vi "Main.vi"() -> ()   [LabVIEW 2025]
doc: "This template is for the Queued Message Handler design pattern.\n\nThe Event Handling Loop generates messages based on user interface actions.\n\nThe Message Handling Loop processes messages generated by the Event Handling Loop, or by other messages. The messages are string values, so new messages can be added easily to the Message Cases case structure in the Message Handling Loop. Each message cluster can also provide an optional value for Message Data, which is a variant that can be converted to whatever message-specific data is required."
uses:
  Public/Controls/CCW button.ctl
  Public/Controls/CW button.ctl
  controls/UI Data.ctl
  support/Message Queue/Enqueue Message (Single).vi
  <vilib>/Utility/error.llb/Error Cluster From Error Code.vi
  <vilib>/ErrorRing/Error Ring.xnode
  support/Message Queue/Message Queue.lvlib
  support/User Event - Stop/User Event - Stop.lvlib
  NI_DAQ/Libraries/NI DAQ/NI DAQ.lvlib
panel:
  in  "Read sensor":bool
  in  "Exit":bool
  in  "Go to zero":bool
  in  "Set zero":bool
  out "Ready":bool caption="Arduino ready"
  out "Save":bool caption="Guardando datos"
  out "Angulo M2":dbl caption="Ángulo \nActual M2" format="%#_3g°"
  out "Angulo M1":dbl caption="Ángulo \nActual M1" format="%#_3g°"
  out "0° M2":bool
  out "0° M1":bool
  in  "RESOLUCIÓN":dbl=1.0 caption="Avance" format="%#_g°"
  in  "CW Button M1":T1
  in  "CCW Button M1":T2
  in  "CCW Button M2":T1
  in  "CW Button M2":T2
  in  "Tab Control":T3(tab)
  out "Valor de Sensor":dbl(slide) scale=0.0..1.0
  in  "Intensidad del Láser":u8(slide) step=1 scale=0.0..255.0
  out "Real Time Measurement":cluster{"X":dbl, "Y":dbl}[](graph)
  in  "Ángulo final":dbl=90.0
  in  "Move motors":bool
  in  "Tiempo (segundos)":dbl=600.0
  in  "Init Fixed Angle":bool
  out "Valor de Sensor 2":dbl(slide) caption="Valor de Sensor" scale=0.0..1.0
  out "Real Time Measurement 2":cluster{"X":dbl, "Y":dbl}[](graph)
  in  "Realizar Análisis":bool
  in  "Abrir Archivo":path
  in  "q Final":dbl=80.0
  in  "q Inicial":dbl=40.0
  out "No. de Muestras":i32
  out "Ancho de Curva":dbl format="%#.3g"
  out "Intensidad \nMáxima":dbl
  out "qR":dbl
  out "Intensidad \nMínima":dbl
  out "q Medio":dbl
  out "Brewster Angle Analysis":cluster{"EJE X":dbl[], dbl[]}(graph)
  out "Índice":dbl
  in  "Abeles Brewster":bool
  in  "Abrir Archivo de Sustrato":path
  in  "Abrir Archivo de Película":path
  in  "calcular error":bool
  out "Abeles Brewster Analysis":cluster{dbl[], dbl[]}[](graph)
  in  "q Inicial 2":dbl=40.0
  in  "q Final  2":dbl=80.0
  out "Película qB":dbl
  out "Película qB +error":dbl
  in  "Error (Grados)":dbl
  out "Sustrato qB":dbl
  out "Sustrato IR":dbl format="%#.4g"
  out "Película IR":dbl format="%#.4g"
  out "ángulo B medio":dbl
  out "Película IR +error":dbl format="%#.4g"
  in  "Cero Maquina":bool
  out "Idle":bool
  in  "Stop motors":bool
  # "Programa: Control de motores a pasos \npara medición de ángulo de Brewster y \ntécnica de Abelès-Brewster"
  # "Desarrollado por: Oscar Javier Silva Hernández &\nDiego Torres Armenta"
  # "Controles Manuales y Automáticos"
  # "MOTOR 1"
  # "MOTOR 2"
  # "Información del sistema"
  # "¡ATENCIÓN! Lea estas instrucciones y recomendaciones antes de operar el programa.\nEste programa ejecuta el control manual y automático del sistema en general.\nUna vez que se haya elegido el puerto COM donde tenemos ubicada nuestra tarjeta de adquisición de datos, el programa inicializará con un protocolo de calibración de motores. NO PRESIONE NINGÚN BOTÓN.\nDe manera automática el programa moverá las platinas rotatorias al ángulo 0°. Una vez que los indicadores 0° M1 y 0° M2 estén encendidos, el indicador del Ángulo Actual M1 se habilitará y el podremos iniciar a operar el programa."
  # "Controles Manuales y Automáticos (Controladores e Indicadores)\n\n-MOTOR 1 & 2: Para ambos motores se tiene un botón de movimiento hacia adelante y otro botón de movimiento hacia atrás indicado con flechas. Durante el reinicio de posición 0°, el botón hacia atrás se deshabilita para evitar conflictos mecánicos.\n-0° M1 & 0° M2: Indicadores de posición 0° para ambos motores.\n-FIN: Indica si se está terminó de realizar un movimiento.\n-Ángulo Actual M1 & M2: Muestra la posición actual para cada motor.\n-RESOLUCIÓN: Valor de grados definido por el usuario para realizar movimientos manuales de manera independiente para cada motor. Es utilizado para alinear el sistema con respecto al láser antes y después de realizar mediciones.\n-Reiniciar Posición: Inicia el protocolo de reinicio de posición para regresar los motores a 0°.\n-Mover y Guardar: Se inicia el barrido ángular desde la posición actual de los motores hasta la posición indicada en el controlador Barrido Angular.\n-Cancelar: Cancela cualquier movimiento o instrucción que se esté ejecutando. My útil para detener instrucciones y cerrar el programa sin tener conflictos."
  # "Parámetros iniciales & Información (Controladores e Indicadores)\n\n-SALIR: Cerramos el programa una vez que hayamos terminado de utilizarlo. Es importante no presionar este botón en medio de un movimiento de motor o alguna otra instrucción.\n-Pantalla: Toda la información generada por los eventos de usuario es mostrada en esta pantalla.\n-Programa habilitado: Se enciende cuando el proceso de inicialización se realiza exitosamente y el programa queda listo para operar.\n-Guardar Datos: Indica si los datos están siendo capturados durante el barrido angular."
  # "Gráfica, Ángulo de Brewster & Abelès-Brewster Analysis\n\n-Gráfica: Esta sección es utilizada para llevar a cabo las mediciones. Dentro podemos encontrar un indicador del valor de la intensidad de la luz capturada por el sensor, un controlador para la intensidad de la luz de salida del láser semiconductor.\n-Ángulo de Brewster: En esta sección podemos realizar el análisis de ángulo de Brewster de mediciones realizadas por el sistema para encontrar los parámetros característicos de la curva. Seleccionamos el archivo deseado, definimos el ángulo inicial y final y presionamos el botón ANALISIS.\n-Abelès-Brewster: Muy similar a la sección anterior, podemos realizar el ánalisis de Abelès-Brewster de mediciones realizadas para sustratos con y sin película delgada. También podemos calcular el error del resultado."
  # "Montura de\nSustratos"
  # "Ensamble \nde Motores"
  # "Montura \nde Prismas"
  # "Sistema Completo con Montura de Sustratos"
  # "Ensamble de Láser con Polarizador"
  # "Sistema Completo con Montura de Prismas"
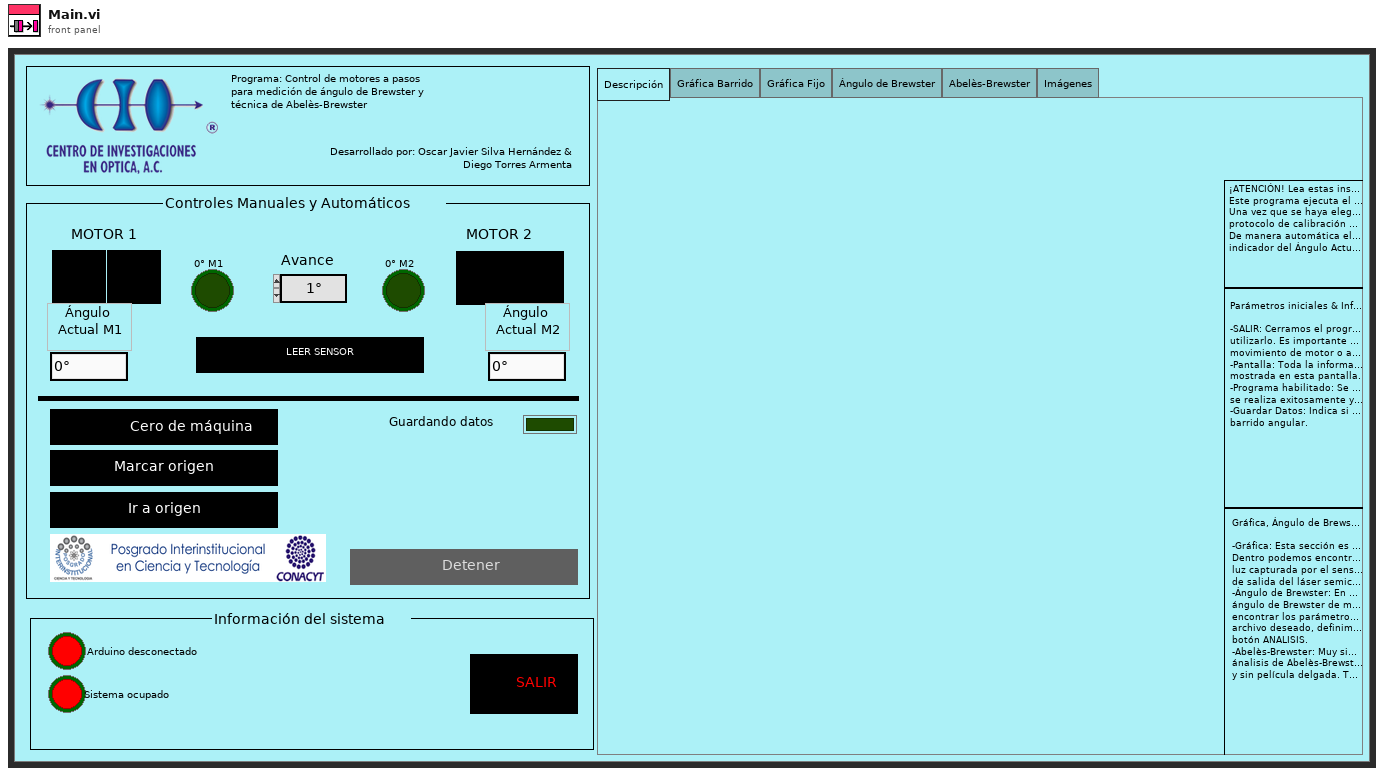
[diagram p1: front panel]
types:
  T1 = typedef "CW button.ctl" = bool
  T2 = typedef "CCW button.ctl" = bool
  T3 = enum32{"Descripción", "Gráfica Barrido", "Gráfica Fijo", "Ángulo de Brewster", "Abelès-Brewster", "Imágenes"}
  T4 = typedef "UI Data.ctl" = cluster{"Exit":refnum<vi>, "DAQ Module ID":i32}
  T5 = typedef "NI DAQ.lvlib/Broadcast Events--cluster.ctl" = cluster{"Module Did Init":refnum<user-event>, "Status Updated":refnum<user-event>, "Error Reported":refnum<user-event>, "Module Did Stop":refnum<user-event>, "Update Module Execution Status":refnum<user-event>, "Digital data acquired":refnum<user-event>, "Device connected":refnum<user-event>, "Connection failed":refnum<user-event>, "Analog data acquired":refnum<user-event>}
  T6 = typedef "Message Queue.lvlib/All Message Queues.ctl" = cluster{"UI":refnum<queue>}
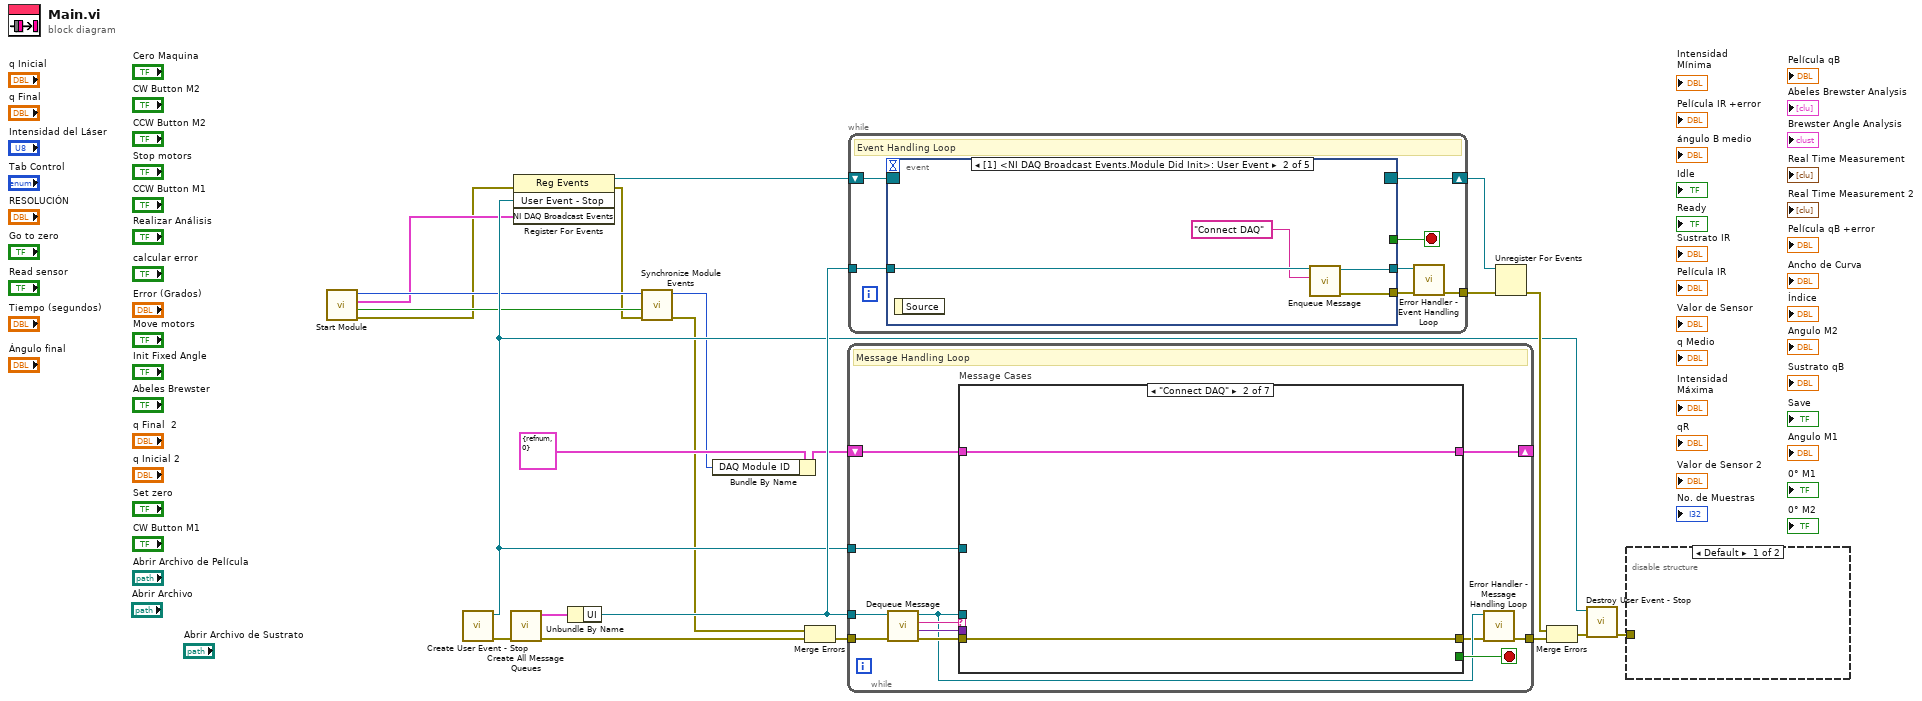
[diagram p0: block diagram]
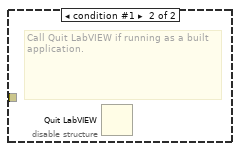
[diagram p2: hidden frame]
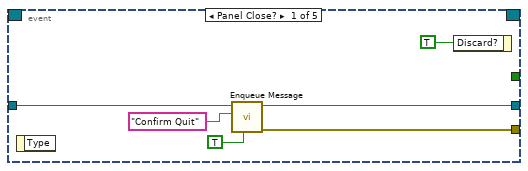
[diagram p3: hidden frame]
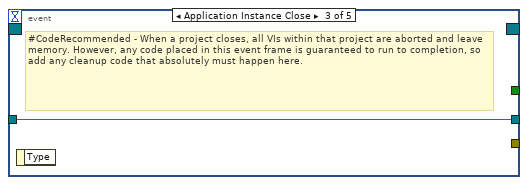
[diagram p4: hidden frame]
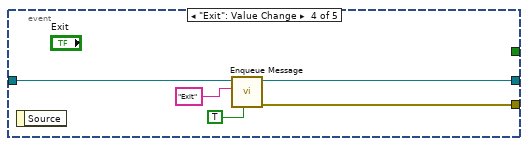
[diagram p5: hidden frame]
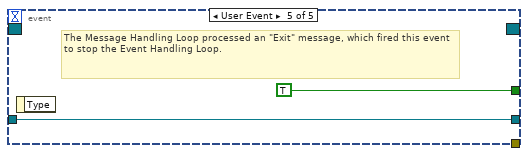
[diagram p6: hidden frame]
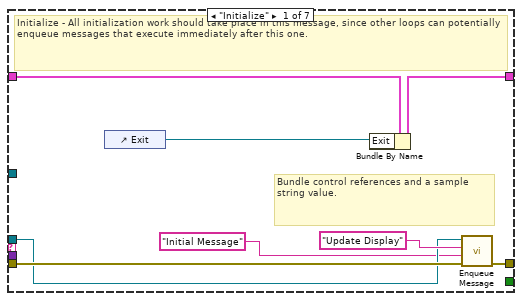
[diagram p7: hidden frame]
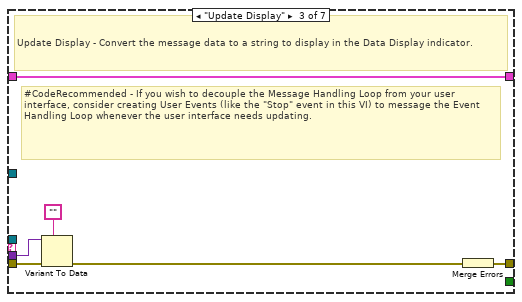
[diagram p8: hidden frame]
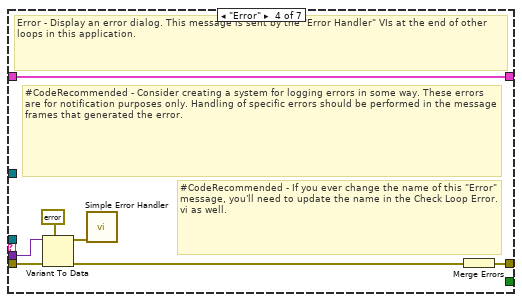
[diagram p9: hidden frame]
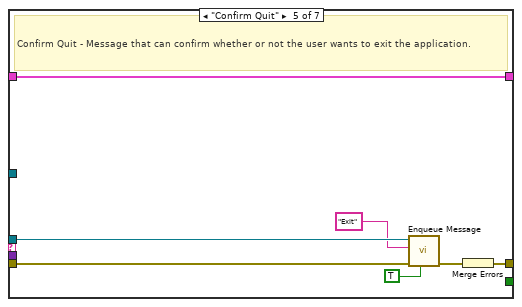
[diagram p10: hidden frame]
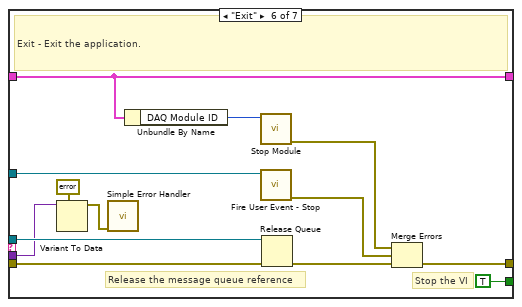
[diagram p11: hidden frame]
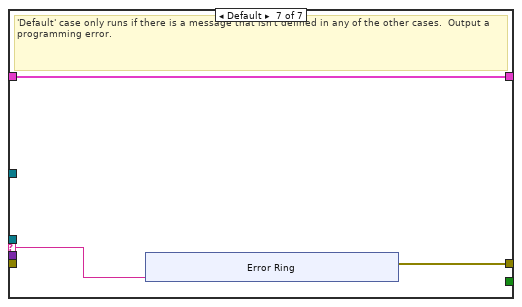
[diagram p12: hidden frame]
diagram:
  n1 = call "Start Module.vi"() -> ("error out"=w5:errorcluster, "Wait for Event Sync?"=w7:bool, "NI DAQ Broadcast Events"=w6:T5, "Module ID"=w8:i32)  [unwired: 8 in]
  n2 = call "Create User Event - Stop.vi"() -> ("error out"=w18:errorcluster, "User Event - Stop"=w10:refnum<user-event>)  [unwired: 10 in]
  n3 = call "Create All Message Queues.vi"("error in (no error)"=w18) -> ("error out"=w22:errorcluster, "Message Queues out"=w21:T6)  [unwired: 9 in]
  n4 = register-events(error in=w5, w10, w6) -> (reference out=w11:refnum<event-registration>, error out=w4:errorcluster)  [unwired: 1 in]
  n5 = Unbundle By Name(w21) -> ("UI"=w19:refnum<queue>)
  n6 = call "Synchronize Module Events.vi"("error in"=w4, "Wait for Event Sync?"=w7, "Module ID in"=w8) -> ("error out"=w3:errorcluster, "Module ID out"=w1:i32)  [unwired: 7 in]
  n7 = Bundle By Name(cluster=T4 {"Exit"=refnum, "DAQ Module ID"=0} ("Data Cluster"), "DAQ Module ID"=w1) -> (w2:T4)
  n8 = Merge Errors(w3, w22) -> (w9:errorcluster)
  n9 = while {
    tunnel: w19 -> [w26]
    shift-right: [w33] -> _
    shift-left: w2 -> [w34]
    tunnel: w10 -> [w31]
    tunnel: w9 -> [w30]
    tunnel: [w24] -> w20
    stop <- w32 stop-if-true
    # "Message Handling Loop"
    n10 = call "Dequeue Message.vi"("error in (no error)"=w30, "Message Queue"=w26) -> ("error out"=w29:errorcluster, "Message Data"=w27:variant, "Message"=w28:string, "dup Message Queue"=w25:refnum<queue>)  [unwired: 6 in]
    n11 = case "Message Cases" shown="\"Connect DAQ\"" w28 {
      selector: w28 -> [_ _ _ _ _ _ w78]
      tunnel: w25 -> [w37 _ _ _ w60 w77 _]
      tunnel: w29 -> [w41 w44 w48 w57 w64 w71 _]
      tunnel: [w42 w44 w49 w51 w62 w74 w79] -> w23
      tunnel: w34 -> [w40 w43 w50 w56 w63 w67 w80]
      tunnel: [w39 w43 w50 w56 w63 w67 w80] -> w33
      tunnel: [_ _ _ _ _ TRUE _] -> w32
      tunnel: w27 -> [_ _ w47 w55 _ w68 _]
      tunnel: w31 -> [_ _ _ _ _ w73 _]
      frame "Initialize" {
        # "Bundle control references and a sample string value."
        # "Initialize - All initialization work should take place in this message, since other loops can potentially enqueue messages that execute immediately after this one."
        n12 = control-ref of="Exit"() -> (w35:refnum<vi>)
        n13 = Bundle By Name(cluster=w40, "Exit"=w35) -> (w39:T4)
        n14 = call-poly "Enqueue Message.vi"("error in (no error)"=w41, "Message Data"="Initial Message" ("Initial Message"), "Message"="Update Display", "Message Queue"=w37) -> ("error out"=w42:errorcluster)  [unwired: 6 in, 1 out]
      }
      frame "Connect DAQ" {
      }
      frame "Update Display" {
        # "#CodeRecommended - If you wish to decouple the Message Handling Loop from your user interface, consider creating User Events (like the \"Stop\" event in this VI) to message the Event Handling Loop whenever the user interface needs updating."
        # "Update Display - Convert the message data to a string to display in the Data Display indicator."
        n15 = Variant To Data(error in=w48, type="", Variant=w47) -> (error out=w45:errorcluster)  [unwired: 1 out]
        n16 = Merge Errors(w45) -> (w49:errorcluster)
      }
      frame "Error" {
        # "#CodeRecommended - If you ever change the name of this \"Error\" message, you'll need to update the name in the Check Loop Error.vi as well."
        # "#CodeRecommended - Consider creating a system for logging errors in some way. These errors are for notification purposes only. Handling of specific errors should be performed in the message frames that generated the error."
        # "Error - Display an error dialog. This message is sent by the \"Error Handler\" VIs at the end of other loops in this application."
        n17 = Variant To Data(error in=w57, type=errorcluster {"status"=FALSE, "code"=0, "source"=""} ("error constant"), Variant=w55) -> (data=w53:errorcluster, error out=w52:errorcluster)
        n18 = call <vilib>:"Simple Error Handler.vi"("error in (no error)"=w53) -> ()  [unwired: 4 in, 5 out]
        n19 = Merge Errors(w52) -> (w51:errorcluster)
      }
      frame "Confirm Quit" {
        # "Confirm Quit - Message that can confirm whether or not the user wants to exit the application."
        n20 = call-poly "Enqueue Message.vi"("Priority Message? (F)"=TRUE, "error in (no error)"=w64, "Message"="Exit", "Message Queue"=w60) -> ("error out"=w61:errorcluster)  [unwired: 6 in, 1 out]
        n21 = Merge Errors(w61) -> (w62:errorcluster)
      }
      frame "Exit" {
        # "Stop the VI"
        # "Release the message queue reference"
        # "Exit - Exit the application."
        n22 = Variant To Data(type=errorcluster {"status"=FALSE, "code"=0, "source"=""} ("error constant"), Variant=w68) -> (data=w69:errorcluster)  [unwired: 1 in, 1 out]
        n23 = call <vilib>:"Simple Error Handler.vi"("error in (no error)"=w69) -> ()  [unwired: 4 in, 5 out]
        n24 = Unbundle By Name(w67) -> ("DAQ Module ID"=w66:i32)
        n25 = call "Stop Module.vi"("Module ID"=w66) -> ("error out"=w65:errorcluster)  [unwired: 10 in]
        n26 = call "Fire User Event - Stop.vi"("User Event - Stop"=w73) -> ("error out"=w72:errorcluster)  [unwired: 10 in]
        n27 = Release Queue(queue=w77, error in (no error)=w71) -> (error out=w75:errorcluster)  [unwired: 1 in, 2 out]
        n28 = Merge Errors(w65, w72, w75) -> (w74:errorcluster)
      }
      frame Default {
        # "'Default' case only runs if there is a message that isn't defined in any of the other cases.  Output a programming error."
        n29 = xnode "Error Ring"("parameter 0"=w78) -> ("error out"=w79:errorcluster)
      }
    }
    n30 = call "Error Handler - Message Handling Loop.vi"("error in (no error)"=w23, "Message Queue"=w25) -> ("dup error in"=w24:errorcluster)  [unwired: 8 in, 1 out]
  }
  n31 = while {
    tunnel: w19 -> [w94]
    shift-right: [w92] -> w15
    shift-left: w11 -> [w93]
    tunnel: [w88] -> w12
    stop <- w90 stop-if-true
    # "Event Handling Loop"
    n32 = event shown="[1] <NI DAQ Broadcast Events.Module Did Init>: User Event" {
      selector: w93 -> [_ _ _ _ _]
      dyn-events: [_ _ _ _ _] -> w92
      timeout: _ -> [_ _ _ _ _]
      tunnel: [_ _ _ _ TRUE ("Discard?")] -> w90
      tunnel: w94 -> [w99 w104 w105 w110 w112]
      tunnel: [w98 w102 _ w109 _] -> w91
      tunnel: [w97 w103 w105 w108 w112] -> w89
      event Panel Close? {
        n33 = event-data() -> ()  [unwired: 1 in, 1 out]
        n34 = call-poly "Enqueue Message.vi"("Priority Message? (F)"=TRUE, "Message"="Confirm Quit", "Message Queue"=w99) -> ("error out"=w98:errorcluster, "dup Message Queue"=w97:refnum<queue>)  [unwired: 7 in]
        n35 = event-data("Discard?"=TRUE) -> ()  [unwired: 1 in, 1 out]
      }
      event User Event {
        n36 = event-data() -> ()  [unwired: 1 in, 1 out]
        n37 = call-poly "Enqueue Message.vi"("Message"="Connect DAQ", "Message Queue"=w104) -> ("error out"=w102:errorcluster, "dup Message Queue"=w103:refnum<queue>)  [unwired: 8 in]
      }
      event Application Instance Close {
        # "#CodeRecommended - When a project closes, all VIs within that project are aborted and leave memory. However, any code placed in this event frame is guaranteed to run to completion, so add any cleanup code that absolutely must happen here."
        n38 = event-data() -> ()  [unwired: 1 in, 1 out]
      }
      event "Exit": Value Change {
        n39 = event-data() -> ()  [unwired: 1 in, 1 out]
        n40 = call-poly "Enqueue Message.vi"("Priority Message? (F)"=TRUE, "Message"="Exit", "Message Queue"=w110) -> ("error out"=w109:errorcluster, "dup Message Queue"=w108:refnum<queue>)  [unwired: 7 in]
      }
      event User Event {
        # "The Message Handling Loop processed an \"Exit\" message, which fired this event to stop the Event Handling Loop."
        n41 = event-data() -> ()  [unwired: 1 in, 1 out]
      }
    }
    n42 = call "Error Handler - Event Handling Loop.vi"("error in (no error)"=w91, "Message Queue"=w89) -> ("dup error in"=w88:errorcluster)  [unwired: 8 in, 1 out]
  }
  n43 = Unregister For Events(event registration refnum=w15, error in=w12) -> (error out=w16:errorcluster)
  n44 = Merge Errors(w16, w20) -> (w17:errorcluster)
  n45 = call "Destroy User Event - Stop.vi"("error in (no error)"=w17, "User Event - Stop"=w10) -> ("error out"=w13:errorcluster)  [unwired: 9 in]
  n46 = disable-structure shown="Default" {
    disable-tunnel: w13 -> [_ _]
    frame condition #0 (active) {
    }
    frame condition #1 {
      # "Call Quit LabVIEW if running as a built application."
      n47 = Quit LabVIEW() -> ()  [unwired: 1 in]
    }
  }
